vi "EventDrivenTest.vi"() -> ()   [LabVIEW 2009]
panel:
  out "Clocks Stepped":i32
  in  "file path (use dialog) 2":path
  in  "Step Clock and Measure":bool
  in  "Clocks To Step":dbl
  in  "Step Clock":bool
  in  "Reset":bool
  in  "FPGA IP Address":string
  in  "Connect to FPGA":bool
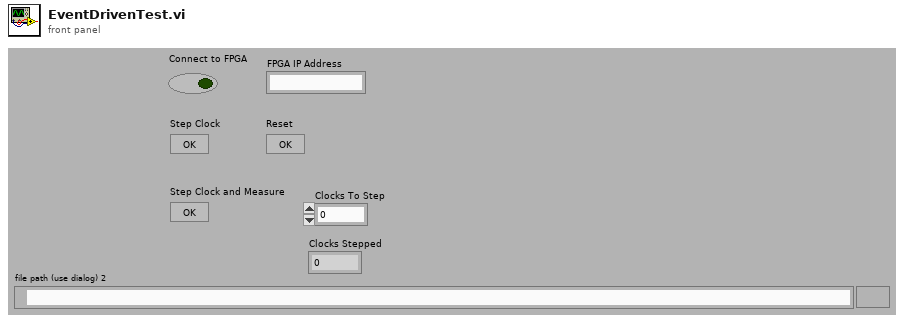
[diagram p1: front panel]
types:
  T1 = enum16{"open", "replace", "create", "open or create", "replace or create", "replace or create with confirmation"}
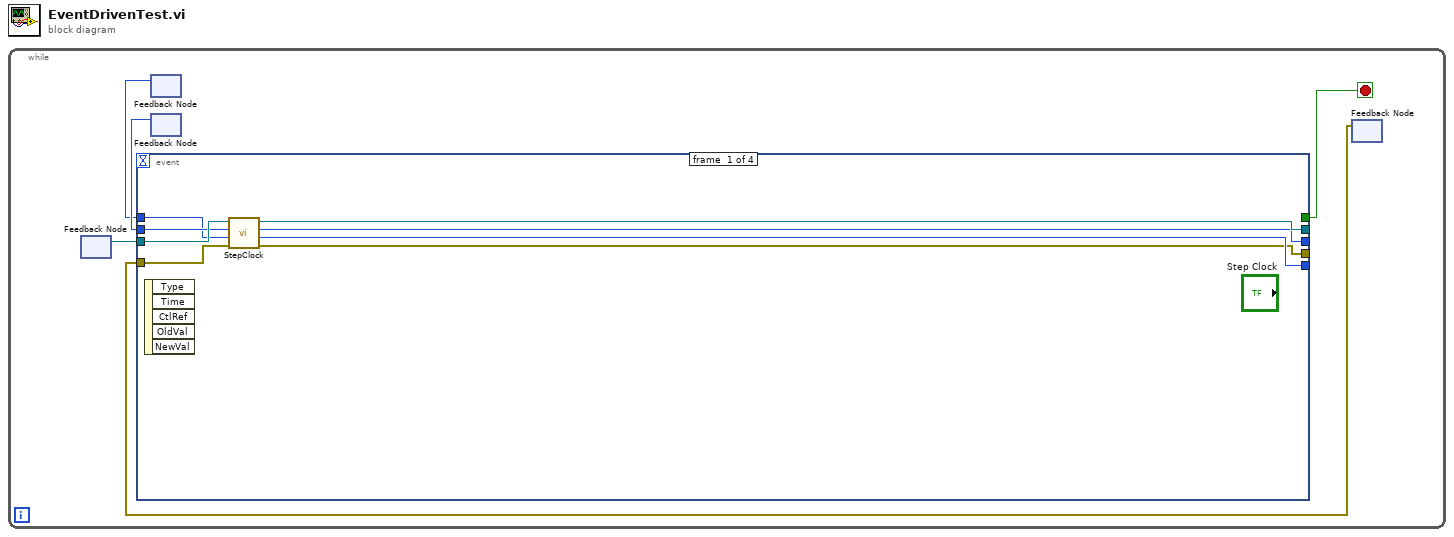
[diagram p0: block diagram]
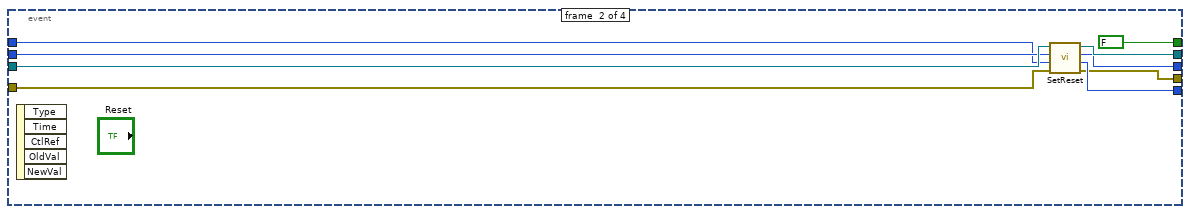
[diagram p2: hidden frame]
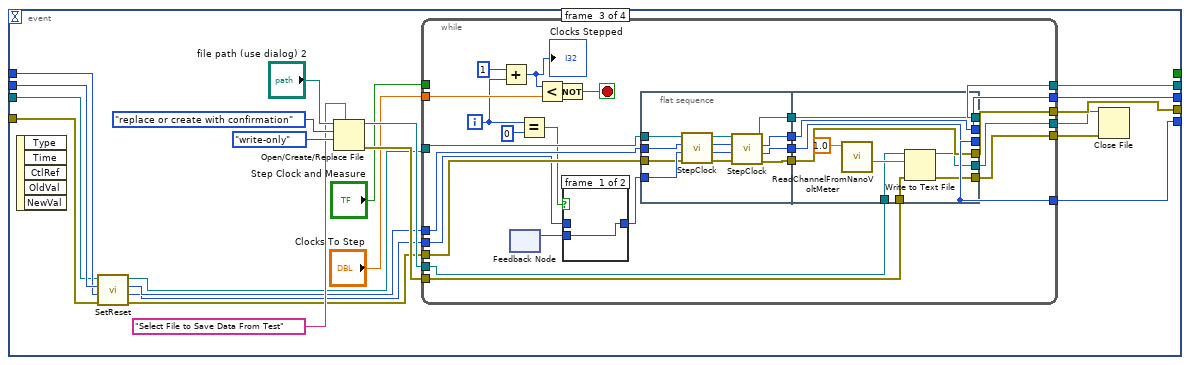
[diagram p3: hidden frame]
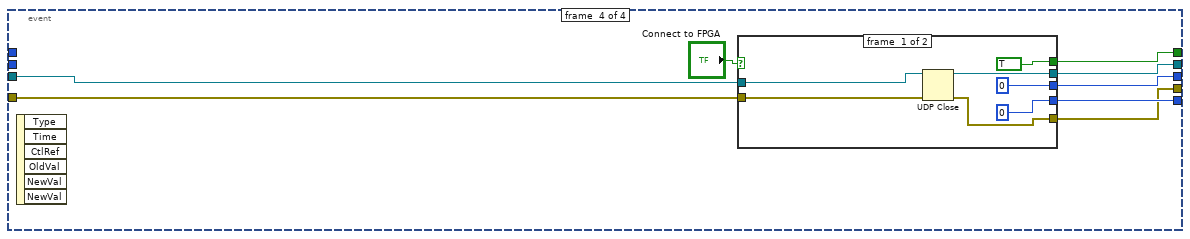
[diagram p5: hidden frame]
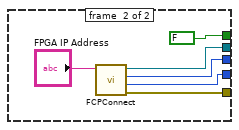
[diagram p6: hidden frame]
diagram:
  n1 = while {
    stop <- w9 stop-if-true
    n2 = feedback #1() -> (w7:refnum<k16>)  [unwired: 1 in]
    n3 = feedback #2() -> (w3:i32)  [unwired: 1 in]
    n4 = feedback #3() -> (w5:u32)  [unwired: 1 in]
    n5 = feedback #4() -> (w1:errorcluster)  [unwired: 1 in]
    n6 = event shown="[2] \"Step Clock and Measure\": Value Change" {
      selector: _ -> [_ _ _ _]
      dyn-events: _ -> [_ _ _ _]
      timeout: _ -> [_ _ _ _]
      tunnel: [_ FALSE _ w105] -> w9
      tunnel: [w13 w21 w48 w104] -> w8
      tunnel: [w12 w20 w47 w103] -> w6
      tunnel: [w11 w19 w27 w102] -> w4
      tunnel: [w10 w18 w46 w101] -> w2
      tunnel: w7 -> [w17 w25 w33 w100]
      tunnel: w5 -> [w16 w24 w35 _]
      tunnel: w3 -> [w15 w23 w34 _]
      tunnel: w1 -> [w14 w22 w32 w99]
      event #0 {
        n7 = event-data() -> ()  [unwired: 1 in, 5 out]
        n8 = call "StepClock.vi"("error in (no error)"=w14, "SequenceNumber"=w15, "address"=w16, "connection ID"=w17) -> ("error out"=w10:errorcluster, "SequenceNumber out"=w11:i32, "address out"=w12:u32, "connection ID out"=w13:refnum<k16>)  [unwired: 4 in]
      }
      event #1 {
        n9 = event-data() -> ()  [unwired: 1 in, 5 out]
        n10 = call "SetReset.vi"("error in (no error)"=w22, "SequenceNumber"=w23, "address"=w24, "connection ID"=w25) -> ("error out"=w18:errorcluster, "SequenceNumber out"=w19:i32, "Address out"=w20:u32, "connection ID out"=w21:refnum<k16>)  [unwired: 4 in]
      }
      event #2 {
        n11 = event-data() -> ()  [unwired: 1 in, 5 out]
        n12 = call "SetReset.vi"("error in (no error)"=w32, "SequenceNumber"=w34, "address"=w35, "connection ID"=w33) -> ("error out"=w28:errorcluster, "SequenceNumber out"=w29:i32, "Address out"=w30:u32, "connection ID out"=w31:refnum<k16>)  [unwired: 4 in]
        n13 = Open/Create/Replace File(file path (use dialog)="file path (use dialog) 2", prompt="Select File to Save Data From Test", operation (0:open)=T1."replace or create with confirmation", access (0:read/write)=enum16{"read/write", "read-only", "write-only"}."write-only") -> (refnum out=w41:refnum<file>, error out=w40:errorcluster)  [unwired: 2 in, 1 out]
        n14 = while {
          tunnel: [w71] -> w48
          tunnel: [w70] -> w47
          tunnel: [w69] -> w46
          tunnel: w41 -> [w68]
          tunnel: w40 -> [w67]
          tunnel: [w66] -> w39
          tunnel: [w65] -> w38
          tunnel: "Step Clock and Measure" -> [_]
          tunnel: "Clocks To Step" -> [w64]
          tunnel: w31 -> [w61]
          tunnel: w30 -> [w60]
          tunnel: w29 -> [w56]
          tunnel: w28 -> [w59]
          tunnel: [w51] -> w27
          i -> [w52]
          stop <- w62 stop-if-true
          n15 = Add(x=1, y=w52) -> (x+y=w50:i32)
          "Clocks Stepped" <- w50
          n16 = feedback #5() -> (w54:i32)  [unwired: 1 in]
          n17 = Equal?(x=w52, y=0) -> (x = y?=w57:bool)
          n18 = Less?(x=w50, y=w64) -> (x < y?=w63:bool)
          n19 = Not(x=w63) -> (.not. x?=w62:bool)
          n20 = case shown="False" w57 {
            tunnel: w56 -> [_ w76]
            tunnel: [w75 w76] -> w55
            tunnel: w54 -> [w75 _]
            frame #0 {
            }
            frame #1 {
            }
          }
          n21 = flat-sequence {
            tunnel: [w78] -> w72
            tunnel: [w79] -> w73
            tunnel: [w80] -> w74
            tunnel: w61 -> [w88]
            tunnel: w60 -> [w87]
            tunnel: w55 -> [w86]
            tunnel: w59 -> [w85]
            tunnel: [w77] -> w49
            tunnel: [w95] -> w69
            tunnel: [w96] -> w51
            tunnel: [w97] -> w70
            tunnel: [w98] -> w71
            tunnel: w74 -> [w95]
            tunnel: w73 -> [w96]
            tunnel: w72 -> [w97]
            tunnel: w68 -> [w92]
            tunnel: w67 -> [w91]
            tunnel: [w90] -> w66
            tunnel: [w89] -> w65
            tunnel: w49 -> [w98]
            frame #0 {
              n22 = call "StepClock.vi"("error in (no error)"=w85, "SequenceNumber"=w86, "address"=w87, "connection ID"=w88) -> ("error out"=w81:errorcluster, "SequenceNumber out"=w82:i32, "address out"=w83:u32, "connection ID out"=w84:refnum<k16>)  [unwired: 4 in]
              n23 = call "StepClock.vi"("error in (no error)"=w81, "SequenceNumber"=w82, "address"=w83, "connection ID"=w84) -> ("error out"=w80:errorcluster, "SequenceNumber out"=w79:i32, "address out"=w78:u32, "connection ID out"=w77:refnum<k16>)  [unwired: 4 in]
            }
            frame #1 {
              n24 = call "ReadChannelFromNanoVoltMeter.vi"("ChannelSelection"=1.0) -> ("String Measurement"=w93:string)  [unwired: 8 in, 2 out]
              n25 = Write to Text File(file (use dialog)=w92, text=w93, error in=w91) -> (refnum out=w90:refnum<file>, error out=w89:errorcluster)  [unwired: 1 in, 1 out]
            }
          }
        }
        n26 = Close File(refnum=w39, error in=w38) -> ()  [unwired: 2 out]
      }
      event #3 {
        n27 = event-data() -> ()  [unwired: 1 in, 6 out]
        n28 = case shown="True" "Connect to FPGA" {
          tunnel: [u32 0 ("FPGA IP Address Out") w118] -> w103
          tunnel: [0 ("Sequence Number") w117] -> w102
          tunnel: [w111 w116] -> w101
          tunnel: [w110 w115] -> w104
          tunnel: [TRUE FALSE] -> w105
          tunnel: w100 -> [w108 _]
          tunnel: w99 -> [w107 _]
          frame #0 {
            n29 = UDP Close(connection ID=w108, 8:w107) -> (connection ID out=w110:refnum<k16>, error out=w111:errorcluster)
          }
          frame #1 {
            n30 = call "FCPConnect.vi"("FPGA IP Address"="FPGA IP Address") -> ("error out"=w116:errorcluster, "Sequence Number"=w117:i32, "FPGA IP Address Out"=w118:u32, "connection ID out"=w115:refnum<k16>)  [unwired: 7 in]
          }
        }
      }
    }
  }
